vi "can_decoder3.vi"() -> ()   [LabVIEW 2015]
panel:
  out "16bit integer":i16
  out "Data":u8[](array[numeric])
  out "time":u32
  out "apv":u8
  out "mcp":u16
  out "vel":dbl
  out "error out":errorcluster
  # "Steering angle"
  # "Steering torque"
  # "RATE?"
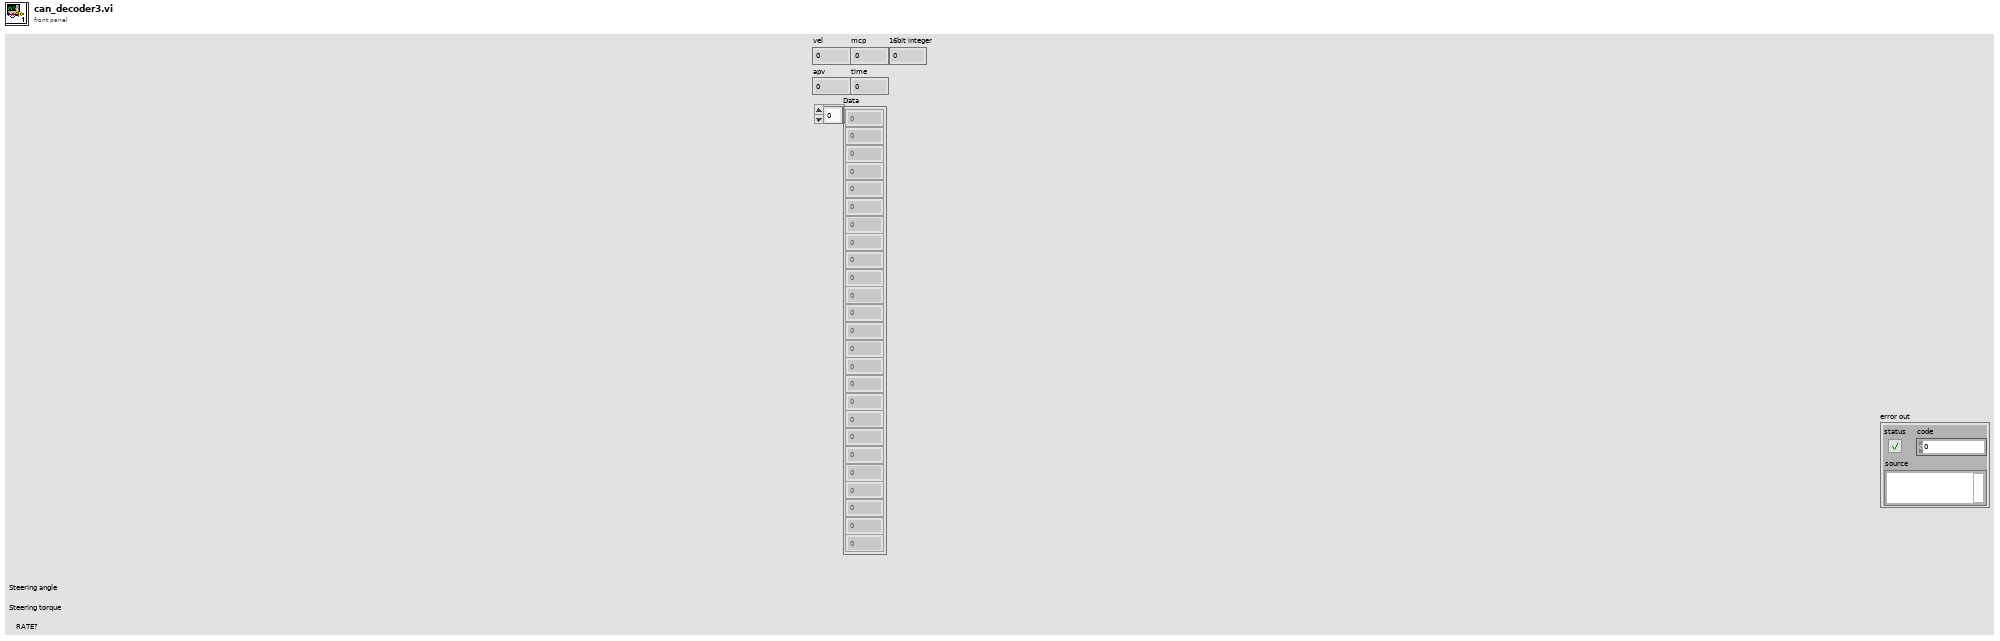
[diagram p1: front panel]
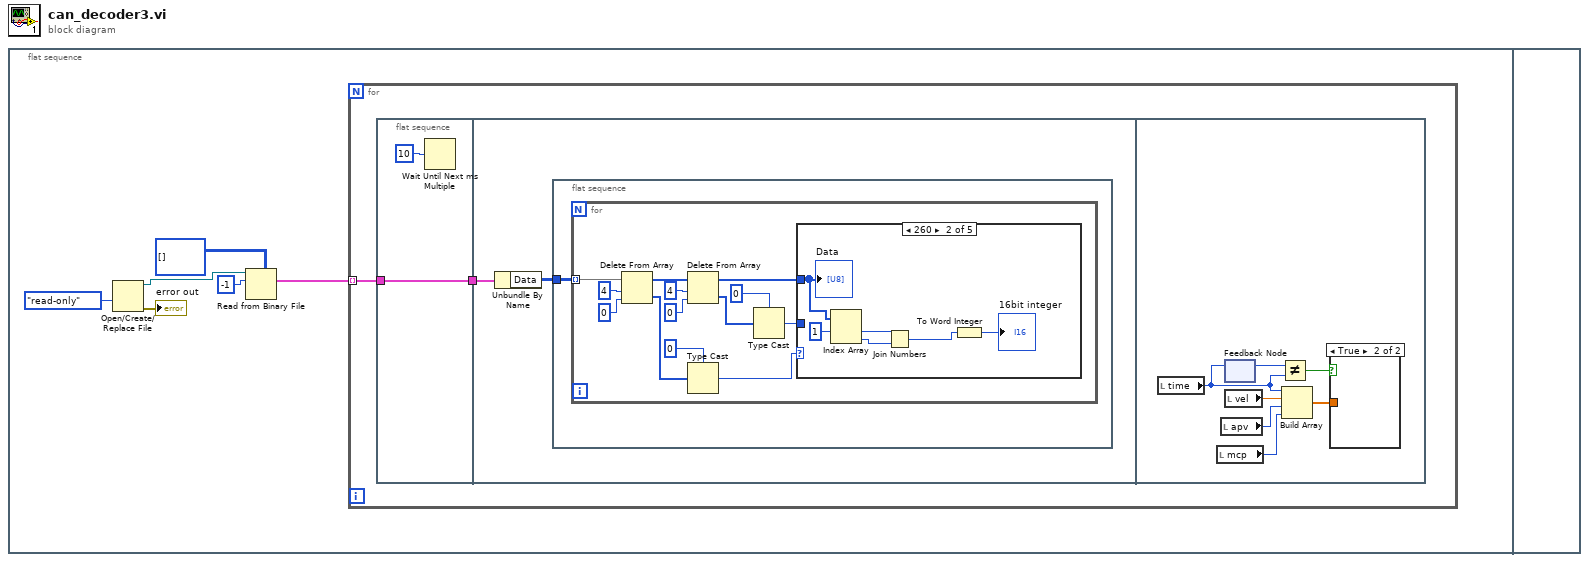
[diagram p0: block diagram]
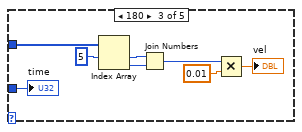
[diagram p3: hidden frame]
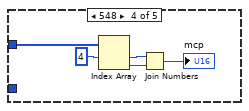
[diagram p4: hidden frame]
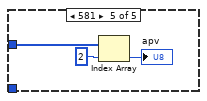
[diagram p5: hidden frame]
diagram:
  n1 = flat-sequence {
    frame #0 {
      n2 = Open/Create/Replace File(access (0:read/write)=enum16{"read/write", "read-only", "write-only"}."read-only") -> (refnum out=w1:refnum<file>, error out=→"error out":errorcluster)  [unwired: 5 in, 1 out]
      n3 = Read from Binary File(5:u8[][] [] ("Data"), 10:-1 ("count (1)"), 11:w1) -> (2:w4:cluster{"Data":u8[][]}[])  [unwired: 3 in, 3 out]
      n4 = for {
        tunnel: w4 -> [w8] mode=indexing
        n5 = flat-sequence {
          tunnel: w8 -> [w10]
          tunnel: [w10] -> w7
          tunnel: w7 -> [w12]
          frame #0 {
            n6 = Wait Until Next ms Multiple(millisecond multiple=u32 10) -> ()  [unwired: 1 out]
          }
          frame #1 {
            n7 = Unbundle By Name(w12) -> ("Data"=w11:u8[][])
            n8 = flat-sequence {
              tunnel: w11 -> [w13]
              frame #0 {
                n9 = for {
                  tunnel: w13 -> [w22] mode=indexing
                  n10 = Delete From Array(array=w22, length=4, index=0) -> (deleted portion=w25:u8[], array with subset deleted=w19:u8[])
                  n11 = Delete From Array(array=w19, length=4, index=0) -> (deleted portion=w15:u8[], array with subset deleted=w17:u8[])
                  n12 = Type Cast(type=u32 0, x=w25) -> (*(type *) &x=w18:u32)
                  n13 = Type Cast(type=u32 0, x=w15) -> (*(type *) &x=w14:u32)
                  n14 = case shown="260" w18 {
                    tunnel: w17 -> [_ w32 w37 w45 w48]
                    tunnel: w14 -> [_ _ w33 _ _]
                    frame 0, Default {
                    }
                    frame 608 {
                      n15 = Index Array(array=w32, index #1=1 ("index")) -> (element #1=w30:u8, element #2=w29:u8)  [unwired: 1 in]
                      n16 = Join Numbers(hi=w30, lo=w29) -> ((hi.lo)=w28:u16)
                      n17 = To Word Integer(number=w28) -> (16bit integer=→"16bit integer":i16)
                      "Data" <- w32
                    }
                    frame 180 {
                      n18 = Index Array(array=w37, index #1=5 ("index")) -> (element #1=w39:u8, element #2=w40:u8)  [unwired: 1 in]
                      n19 = Join Numbers(hi=w39, lo=w40) -> ((hi.lo)=w36:u16)
                      n20 = Multiply(x=w36, y=0.01) -> (x*y=→"vel":dbl)
                      "time" <- w33
                    }
                    frame 548 {
                      n21 = Index Array(array=w45, index #1=4 ("index")) -> (element #1=w43:u8, element #2=w42:u8)  [unwired: 1 in]
                      n22 = Join Numbers(hi=w43, lo=w42) -> ((hi.lo)=→"mcp":u16)
                    }
                    frame 581 {
                      n23 = Index Array(array=w48, index=2) -> (element=→"apv":u8)
                    }
                  }
                }
              }
            }
          }
          frame #2 {
            n24 = local read "time"() -> (w51:u32)
            n25 = local read "mcp"() -> (w53:u16)
            n26 = local read "apv"() -> (w54:u8)
            n27 = feedback-in #1(w51) -> ()
            n28 = feedback #1() -> (w52:u32)  [unwired: 1 in]
            n29 = local read "vel"() -> (w55:dbl)
            n30 = Not Equal?(x=w52, y=w51) -> (x != y?=w50:bool)
            n31 = Build Array(w51, w55, w54, w53) -> (w49:dbl[])
            n32 = case shown="True" w50 {
              tunnel: w49 -> [_ _]
              frame False {
              }
              frame True {
              }
            }
          }
        }
      }
    }
    frame #1 {
    }
  }
